vi "Get LastRoll.vi"(8 "error in (no error)":errorcluster, 11 "Dice in":refnum<class "Dice.lvclass">) -> (0 "error out":errorcluster, 2 "LastRoll":u8, 3 "Dice out":refnum<class "Dice.lvclass">)   [LabVIEW 2016, in "Dice.lvclass"]
uses:
  Dice.lvclass
  Dice.lvclass/Dice.ctl
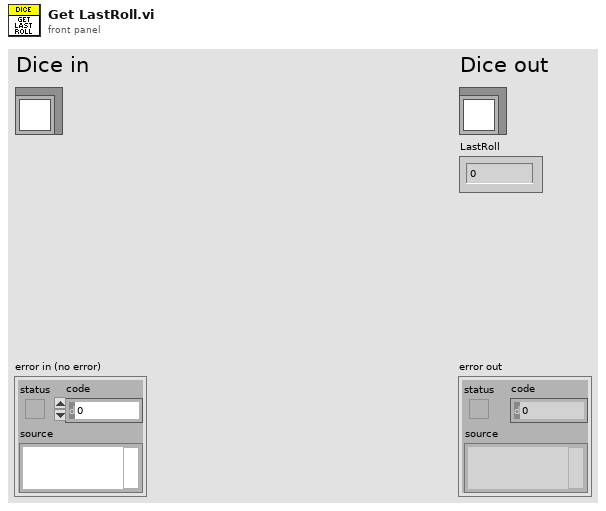
[diagram p1: front panel]
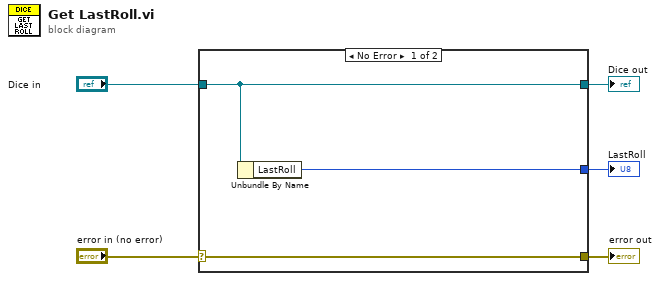
[diagram p0: block diagram]
diagram:
  n1 = case shown="No Error" "error in (no error)" {
    selector: "error in (no error)" -> [w8 w9]
    tunnel: [w8 w9] -> w4
    tunnel: [w7 w10] -> w2
    tunnel: "Dice in" -> [w7 w10]
    tunnel: [w6 _] -> w1
    frame No Error {
      n2 = Unbundle By Name(w7) -> ("LastRoll"=w6:u8)
    }
    frame Error {
    }
  }
  "error out" <- w4
  "Dice out" <- w2
  "LastRoll" <- w1
